vi "Processing_Main.vi"(8 "error in":errorcluster, 11 "QRD":T1) -> (0 "error out":errorcluster)   [LabVIEW 2025]
uses:
  Controls/Queues-Refs-Data.ctl
  Builds/Queue Wrappers.lvlibp/Q Packet.ctl
  Controls/Local Data_Processing.ctl
  Builds/Queue Wrappers.lvlibp
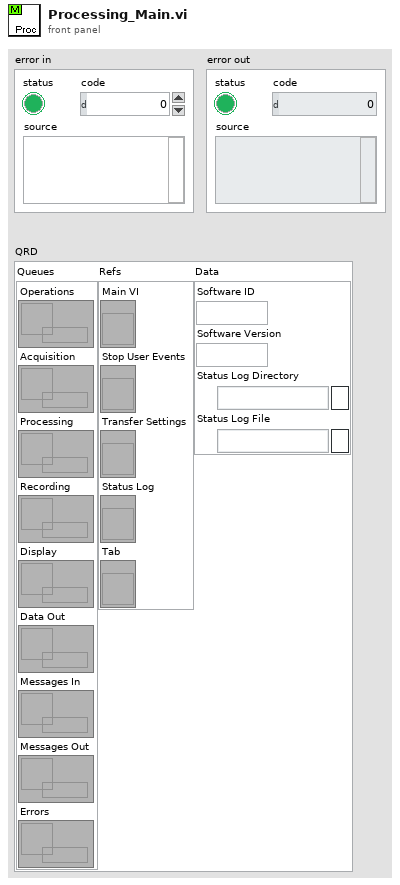
[diagram p1: front panel]
types:
  T1 = typedef "Queues-Refs-Data.ctl" = cluster{"Queues":cluster{"Operations":refnum<queue>, "Acquisition":refnum<queue>, "Processing":refnum<queue>, "Recording":refnum<queue>, "Display":refnum<queue>, "Data Out":refnum<queue>, "Messages In":refnum<queue>, "Messages Out":refnum<queue>, "Errors":refnum<queue>}, "Refs":cluster{"Main VI":refnum<vi>, "Stop User Events":refnum<vi>, "Transfer Settings":refnum<vi>, "Status Log":refnum<vi>, "Tab":refnum<vi>}, "Data":cluster{"Software ID":string, "Software Version":string, "Status Log Directory":path, "Status Log File":path}}
  T2 = typedef "Local Data_Processing.ctl" = cluster{"Loop ID":string}
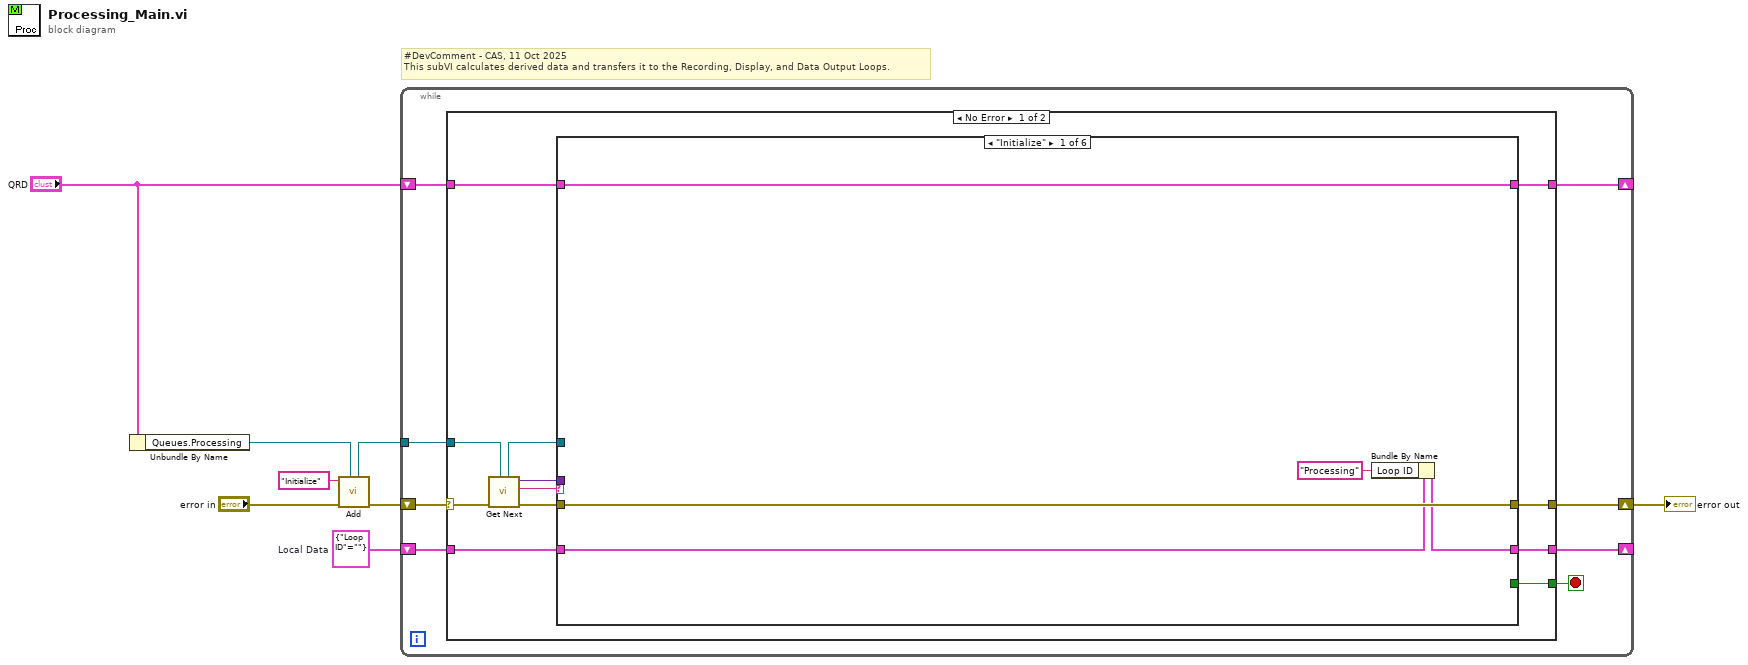
[diagram p0: block diagram]
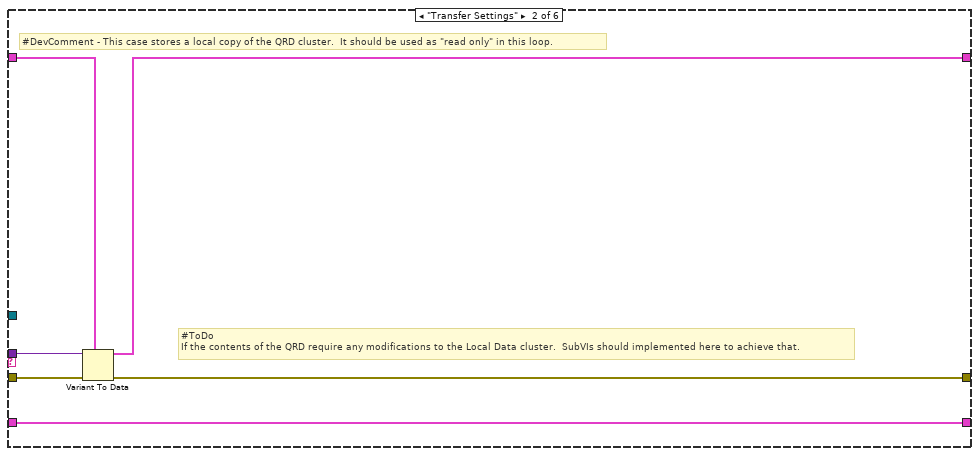
[diagram p2: hidden frame]
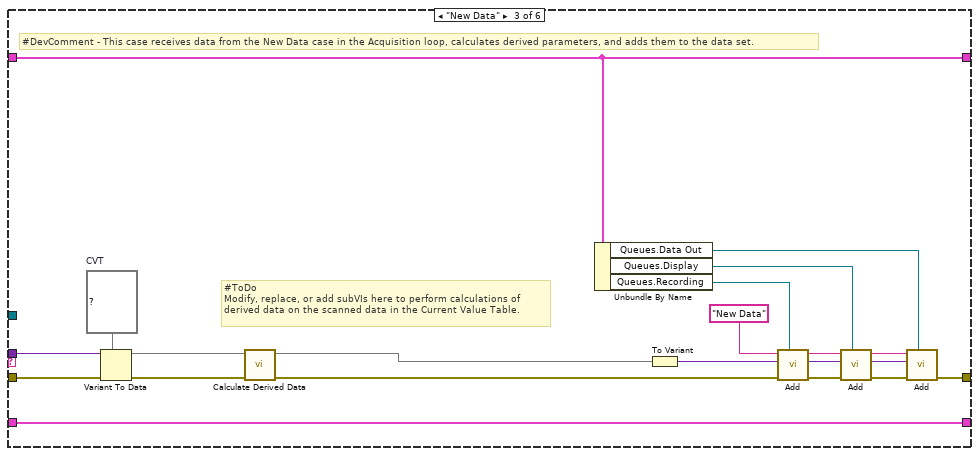
[diagram p3: hidden frame]
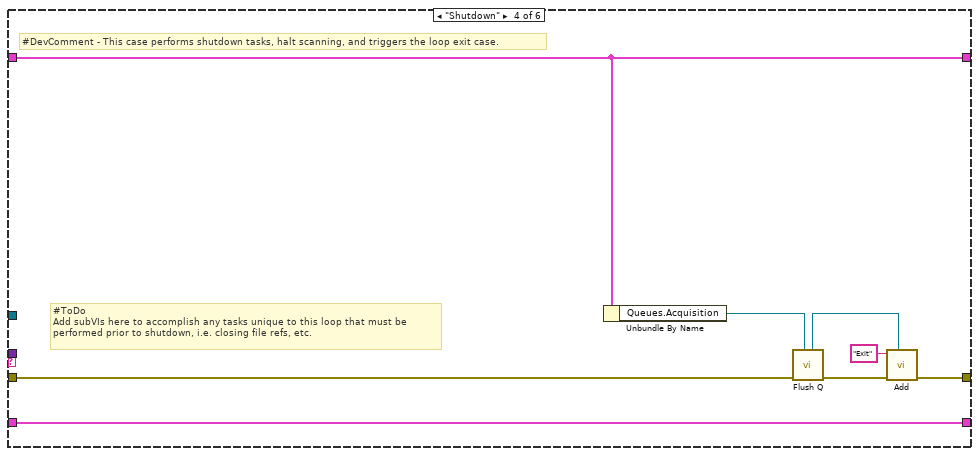
[diagram p4: hidden frame]
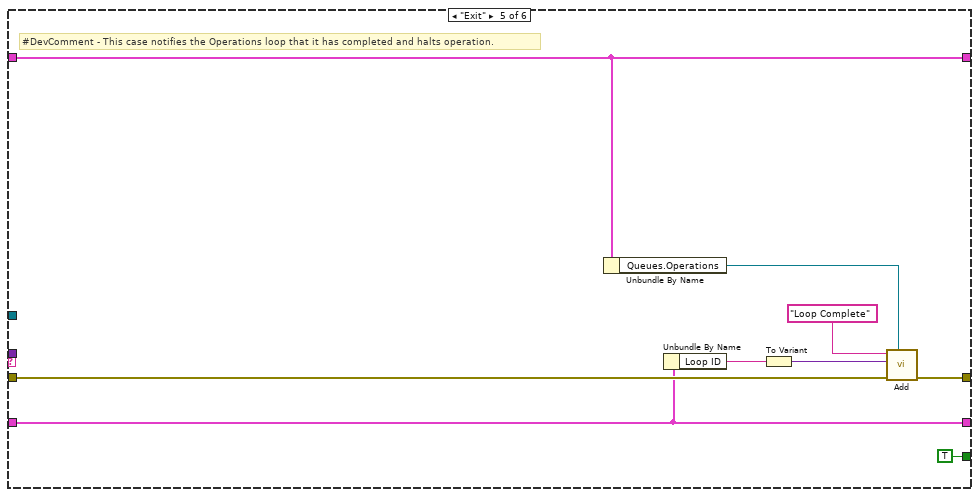
[diagram p5: hidden frame]
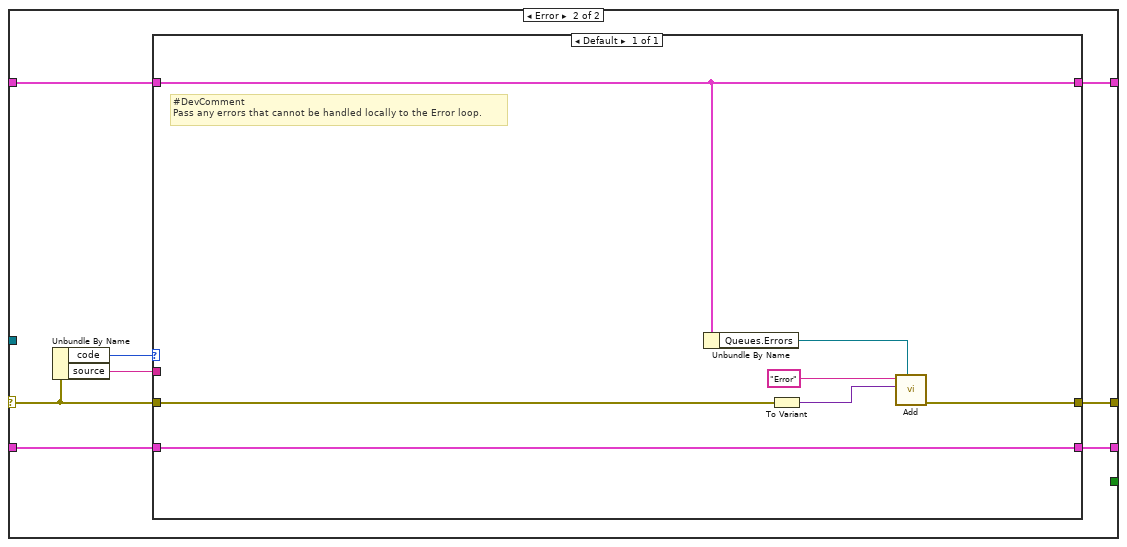
[diagram p7: hidden frame]
diagram:
  w6 = T2 {"Loop ID"=""}  # Local Data
  # "#DevComment - CAS, 11 Oct 2025\nThis subVI calculates derived data and transfers it to the Recording, Display, and Data Output Loops."
  n1 = Unbundle By Name("QRD") -> ("Queues.Processing"=w3:refnum<queue>)
  n2 = call "Add.vi"("Q Ref In"=w3, "error in"="error in", "Packet ID"="Initialize") -> ("error out"=w4:errorcluster, "Q Ref Out"=w2:refnum<queue>)  [unwired: 5 in, 2 out]
  n3 = while {
    shift-right: [w15] -> _
    shift-left: "QRD" -> [w16]
    shift-right: [w13] -> w8
    shift-left: w4 -> [w14]
    tunnel: w2 -> [w12]
    shift-right: [w9] -> _
    shift-left: w6 -> [w11]
    stop <- w10 stop-if-true
    n4 = case shown="No Error" w14 {
      selector: w14 -> [w28 w85]
      tunnel: w16 -> [w25 w82]
      tunnel: [w26 w83] -> w15
      tunnel: [w23 w84] -> w13
      tunnel: w12 -> [w27 _]
      tunnel: w11 -> [w19 w86]
      tunnel: [w18 w81] -> w9
      tunnel: [w17 _] -> w10
      frame No Error {
        n5 = call "Get Next.vi"("Q Ref In"=w27, "error in"=w28) -> ("error out"=w24:errorcluster, "Packet ID"=w20:string, "Payload"=w21:variant, "Q Ref Out"=w22:refnum<queue>)  [unwired: 6 in]
        n6 = case shown="\"Initialize\"" w20 {
          tunnel: [w33 w35 w57 w68 w77 w80] -> w26
          tunnel: w25 -> [w33 w37 w57 w68 w77 w80]
          tunnel: w24 -> [w32 w39 w60 w65 w74 w79]
          tunnel: [w32 w36 w42 w67 w76 w79] -> w23
          tunnel: w22 -> [_ _ _ _ _ _]
          tunnel: w21 -> [_ w38 w59 _ _ _]
          tunnel: w19 -> [w30 w34 w49 w61 w72 w78]
          tunnel: [w31 w34 w49 w61 w72 w78] -> w18
          tunnel: [_ _ _ _ TRUE _] -> w17
          frame "Initialize" {
            n7 = Bundle By Name(cluster=w30, "Loop ID"="Processing") -> (w31:T2)
          }
          frame "Transfer Settings" {
            # "#ToDo\nIf the contents of the QRD require any modifications to the Local Data cluster.  SubVIs should implemented here to achieve that."
            # "#DevComment - This case stores a local copy of the QRD cluster.  It should be used as \"read only\" in this loop."
            n8 = Variant To Data(error in=w39, type=w37, Variant=w38) -> (data=w35:T1, error out=w36:errorcluster)
          }
          frame "New Data" {
            w58 = map{string, string} {}  # CVT
            # "#ToDo\nModify, replace, or add subVIs here to perform calculations of\nderived data on the scanned data in the Current Value Table."
            # "#DevComment - This case receives data from the New Data case in the Acquisition loop, calculates derived parameters, and adds them to the data set."
            n9 = Variant To Data(error in=w60, type=w58, Variant=w59) -> (data=w52:map{string, string}, error out=w53:errorcluster)
            n10 = call "Calculate Derived Data.vi"("error in"=w53, "CVT"=w52) -> ("error out"=w51:errorcluster, "CVT Out"=w50:map{string, dbl})  [unwired: 8 in]
            n11 = Unbundle By Name(w57) -> ("Queues.Data Out"=w40:refnum<queue>, "Queues.Display"=w41:refnum<queue>, "Queues.Recording"=w56:refnum<queue>)
            n12 = To Variant(anything=w50) -> (Variant=w54:variant)
            n13 = call "Add.vi"("Q Ref In"=w56, "error in"=w51, "Payload"=w54, "Packet ID"="New Data") -> ("error out"=w48:errorcluster, "Payload Out"=w46:variant, "Packet ID Out"=w47:string)  [unwired: 4 in, 1 out]
            n14 = call "Add.vi"("Q Ref In"=w41, "error in"=w48, "Payload"=w46, "Packet ID"=w47) -> ("error out"=w43:errorcluster, "Payload Out"=w45:variant, "Packet ID Out"=w44:string)  [unwired: 4 in, 1 out]
            n15 = call "Add.vi"("Q Ref In"=w40, "error in"=w43, "Payload"=w45, "Packet ID"=w44) -> ("error out"=w42:errorcluster)  [unwired: 4 in, 3 out]
          }
          frame "Shutdown" {
            # "#ToDo\nAdd subVIs here to accomplish any tasks unique to this loop that must be\nperformed prior to shutdown, i.e. closing file refs, etc."
            # "#DevComment - This case performs shutdown tasks, halt scanning, and triggers the loop exit case."
            n16 = Unbundle By Name(w68) -> ("Queues.Acquisition"=w63:refnum<queue>)
            n17 = call "Flush Q.vi"("Q Ref In"=w63, "error in"=w65) -> ("error out"=w64:errorcluster, "Q Ref Out"=w62:refnum<queue>)  [unwired: 8 in]
            n18 = call "Add.vi"("Q Ref In"=w62, "error in"=w64, "Packet ID"="Exit") -> ("error out"=w67:errorcluster)  [unwired: 5 in, 3 out]
          }
          frame "Exit" {
            # "#DevComment - This case notifies the Operations loop that it has completed and halts operation."
            n19 = Unbundle By Name(w77) -> ("Queues.Operations"=w73:refnum<queue>)
            n20 = Unbundle By Name(w72) -> ("Loop ID"=w71:string)
            n21 = To Variant(anything=w71) -> (Variant=w70:variant)
            n22 = call "Add.vi"("Q Ref In"=w73, "error in"=w74, "Payload"=w70, "Packet ID"="Loop Complete") -> ("error out"=w76:errorcluster)  [unwired: 4 in, 3 out]
          }
          frame Default {
          }
        }
      }
      frame Error {
        n23 = Unbundle By Name(w85) -> ("code"=w88:i32, "source"=w87:string)
        n24 = case shown="Default" w88 {
          tunnel: w87 -> [_]
          tunnel: w86 -> [w95]
          tunnel: [w95] -> w81
          tunnel: w85 -> [w90]
          tunnel: [w92] -> w84
          tunnel: [w91] -> w83
          tunnel: w82 -> [w91]
          frame Default {
            # "#DevComment\nPass any errors that cannot be handled locally to the Error loop."
            n25 = Unbundle By Name(w91) -> ("Queues.Errors"=w93:refnum<queue>)
            n26 = To Variant(anything=w90) -> (Variant=w89:variant)
            n27 = call "Add.vi"("Q Ref In"=w93, "Payload"=w89, "Packet ID"="Error") -> ("error out"=w92:errorcluster)  [unwired: 5 in, 3 out]
          }
        }
      }
    }
  }
  "error out" <- w8
